vi "TimeSyncServ_Exec.vi"(8 "error in (no error)":errorcluster) -> ()   [LabVIEW 2019, in "PhotonVisionLib.lvlib"]
doc: "Execute a PhotonVision Time Sync Server. It listens for UDP requests from PhotonVision devices and responds with the current FPGA time.\n\nThis VI contains a loop. Do not place this in another loop.\n\nPlace this all by itself in Periodic Tasks.\n\n\nInputs:\n -- Error In -- Optional error input cluster.\n\nOutputs:\n -- <None>"
uses:
  PhotonVisionLib.lvlib
  <vilib>/Rock Robotics/WPI/ThirdParty/JAS_Junk/TrajLib/Trajectory_Library.lvlib
  PhotonVision_Globals.vi
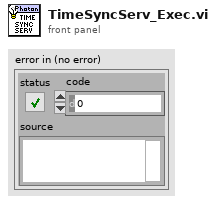
[diagram p1: front panel]
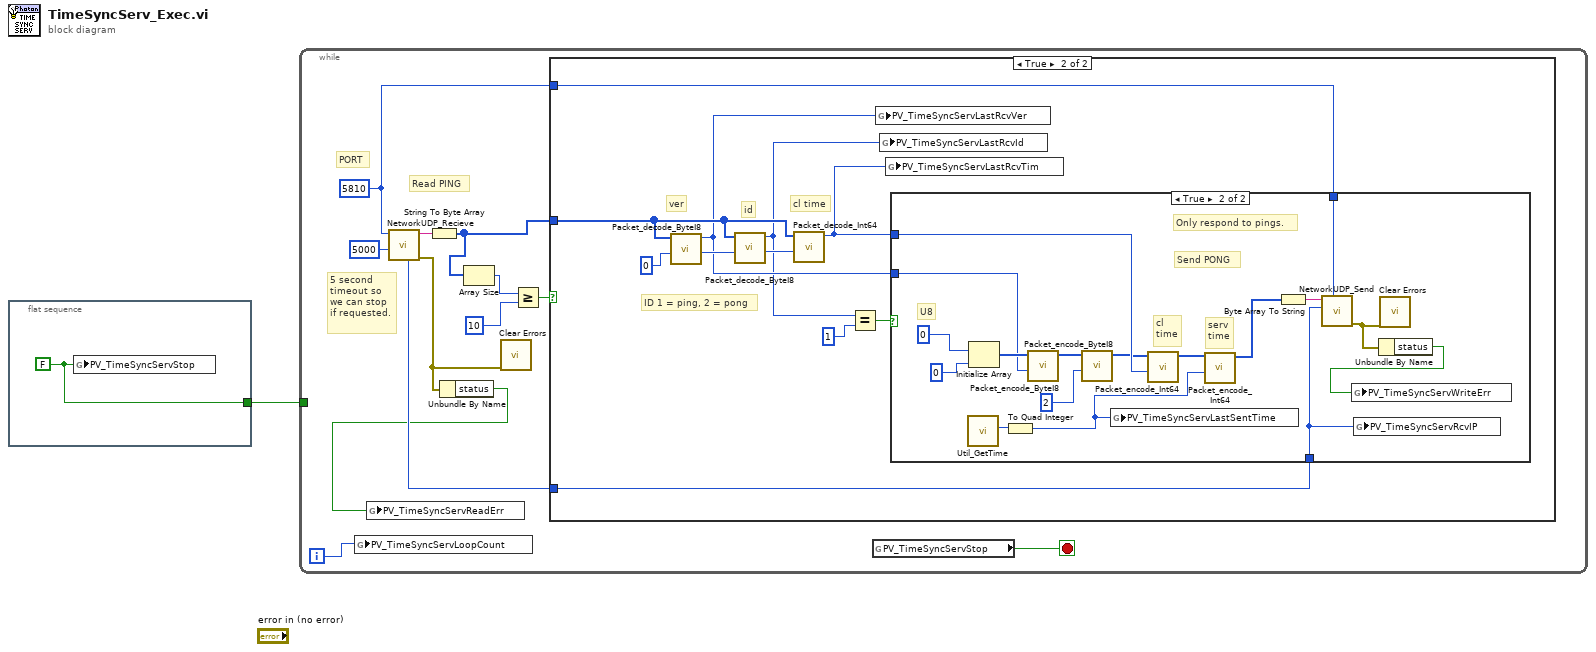
[diagram p0: block diagram]
diagram:
  n1 = flat-sequence {
    tunnel: [w2] -> w1
    frame #0 {
      w2 = FALSE ("PV_TimeSyncStopServ")
      n2 = global write "PhotonVision_Globals.vi" "PV_TimeSyncServStop"(w2) -> ()
    }
  }
  n3 = while {
    tunnel: w1 -> [_]
    i -> [w5]
    stop <- w6 stop-if-true
    w14 = u16 5810 ("receiver port")
    # "Read PING"
    # "PORT"
    # "5 second\ntimeout so\nwe can stop\nif requested."
    n4 = global write "PhotonVision_Globals.vi" "PV_TimeSyncServLoopCount"(w5) -> ()
    n5 = call <vilib>:"NetworkUDP_Recieve.vi"("timeout ms (25000)"=5000, "receiver port"=w14) -> ("error out"=w4:errorcluster, "data out"=w12:string, "SenderAddress"=w8:u32)  [unwired: 5 in, 2 out]
    n6 = String To Byte Array(string=w12) -> (unsigned byte array=w11:u8[])
    n7 = Unbundle By Name(w4) -> ("status"=w3:bool)
    n8 = global write "PhotonVision_Globals.vi" "PV_TimeSyncServReadErr"(w3) -> ()
    n9 = Array Size(array=w11) -> (size(s)=w10:i32)
    n10 = call <vilib>:"Clear Errors.vi"("error in (no error)"=w4) -> ()  [unwired: 5 in, 2 out]
    n11 = Greater Or Equal?(x=w10, y=10) -> (x >= y?=w13:bool)
    n12 = case shown="True" w13 {
      tunnel: w14 -> [_ w23]
      tunnel: w11 -> [_ w22]
      tunnel: w8 -> [_ w21]
      frame False {
      }
      frame True {
        # "ID 1 = ping, 2 = pong"
        # "cl time"
        # "id"
        # "ver"
        n13 = call "Packet_decode_ByteI8.vi"("StartByte"=0, "RawData"=w22) -> ("NextByte"=w24:i32, "Int8_Value"=w18:i8)  [unwired: 8 in]
        n14 = call "Packet_decode_ByteI8.vi"("StartByte"=w24, "RawData"=w22) -> ("NextByte"=w20:i32, "Int8_Value"=w16:i8)  [unwired: 8 in]
        n15 = call "Packet_decode_Int64.vi"("StartByte"=w20, "RawData"=w22) -> ("Int64_Value"=w19:i64)  [unwired: 8 in, 1 out]
        n16 = Equal?(x=w16, y=i8 1) -> (x = y?=w17:bool)
        n17 = global write "PhotonVision_Globals.vi" "PV_TimeSyncServLastRcvVer"(w18) -> ()
        n18 = global write "PhotonVision_Globals.vi" "PV_TimeSyncServLastRcvId"(w16) -> ()
        n19 = global write "PhotonVision_Globals.vi" "PV_TimeSyncServLastRcvTim"(w19) -> ()
        n20 = case shown="True" w17 {
          tunnel: w23 -> [_ w41]
          tunnel: w21 -> [_ w26]
          tunnel: w19 -> [_ w34]
          tunnel: w18 -> [_ w31]
          frame False {
          }
          frame True {
            # "Send PONG"
            # "Only respond to pings."
            # "serv\ntime"
            # "cl\ntime"
            # "U8"
            n21 = call <vilib>:"Util_GetTime.vi"() -> ("FPGA_Time_MicroSeconds"=w28:u64)  [unwired: 9 in, 2 out]
            n22 = Initialize Array(u8 0 ("element"), 0 ("dimension size")) -> (w36:u8[])
            n23 = To Quad Integer(1:w28) -> (0:w27:i64)
            n24 = call "Packet_encode_ByteI8.vi"("Int8_Value"=w31, "RawData In"=w36) -> ("RawData Out"=w42:u8[])  [unwired: 9 in]
            n25 = call "Packet_encode_ByteI8.vi"("Int8_Value"=i8 2, "RawData In"=w42) -> ("RawData Out"=w33:u8[])  [unwired: 9 in]
            n26 = global write "PhotonVision_Globals.vi" "PV_TimeSyncServLastSentTime"(w27) -> ()
            n27 = call "Packet_encode_Int64.vi"("Int64_Value"=w34, "RawData In"=w33) -> ("RawData Out"=w32:u8[])  [unwired: 9 in]
            n28 = call "Packet_encode_Int64.vi"("Int64_Value"=w27, "RawData In"=w32) -> ("RawData Out"=w40:u8[])  [unwired: 9 in]
            n29 = Byte Array To String(unsigned byte array=w40) -> (string=w39:string)
            n30 = call <vilib>:"NetworkUDP_Send.vi"("remote port"=w41, "IP4 Address"=w26, "data string"=w39) -> ("error out"=w30:errorcluster)  [unwired: 6 in, 2 out]
            n31 = global write "PhotonVision_Globals.vi" "PV_TimeSyncServRcvIP"(w26) -> ()
            n32 = Unbundle By Name(w30) -> ("status"=w29:bool)
            n33 = global write "PhotonVision_Globals.vi" "PV_TimeSyncServWriteErr"(w29) -> ()
            n34 = call <vilib>:"Clear Errors.vi"("error in (no error)"=w30) -> ()  [unwired: 5 in, 2 out]
          }
        }
      }
    }
    n35 = global read "PhotonVision_Globals.vi" "PV_TimeSyncServStop"() -> (w6:bool)
  }
